vi "SelectdBaseFilesToRecover_Core.vi"(8 "Description":string="Select Condition Vector Settings To Load", 9 "Files To Recover":string[][](array[string])) -> (3 "Selected Files":string[](array[string]))   [LabVIEW 2011]
panel:
  in  "Cancel":bool caption="Trend to diagram"
  in  "OK":bool caption="Trend to diagram"
  in  "Saved settings":i32[](listbox) caption="Iznosi v èasu RS:"
  out "MP.Status parameters:":string caption="Select Files To Recover"
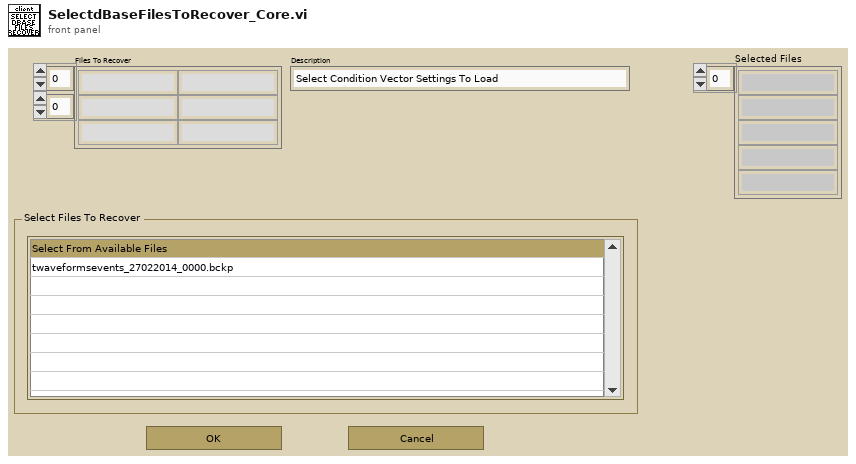
[diagram p1: front panel]
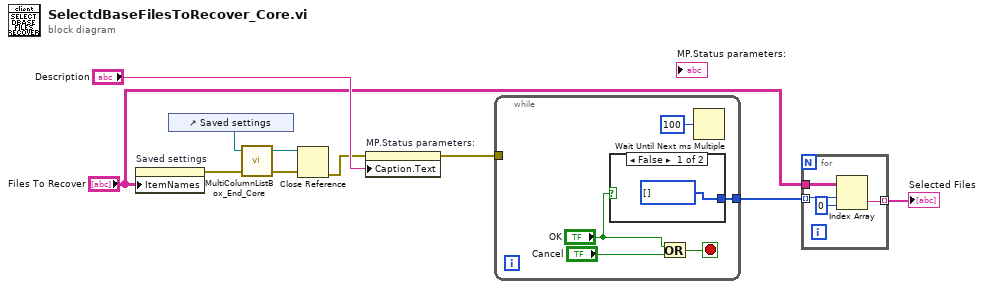
[diagram p0: block diagram]
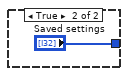
[diagram p2: hidden frame]
diagram:
  n1 = property on="Saved settings" class="MCListbox (strict)"("ItemNames"="Files To Recover") -> (error out=w9:errorcluster)  [unwired: 2 in, 1 out]
  n2 = control-ref of="Saved settings"() -> (w10:refnum<vi>)
  n3 = call "MultiColumnListBox_End_Core.vi"("error in (no error)"=w9, "MCListbox Refnum"=w10) -> ("error out"=w8:errorcluster, "MCListbox Refnum OUT"=w7:refnum<vi>)  [unwired: 2 in]
  n4 = Close Reference(reference=w7, error in (no error)=w8) -> (error out=w5:errorcluster)
  n5 = property on="MP.Status parameters:" class="Str"(error in=w5, "Caption.Text"="Description") -> (error out=w4:errorcluster)  [unwired: 1 in, 1 out]
  n6 = while {
    tunnel: [w15] -> w3
    tunnel: w4 -> [_]
    stop <- w13 stop-if-true
    n7 = case shown="False" "OK" {
      tunnel: [i32[] [] "Saved settings"] -> w15
      frame False {
      }
      frame True {
      }
    }
    n8 = Or(x="OK", y="Cancel") -> (x .or. y?=w13:bool)
    n9 = Wait Until Next ms Multiple(millisecond multiple=u32 100) -> ()  [unwired: 1 out]
  }
  n10 = for {
    tunnel: w3 -> [w19] mode=indexing
    tunnel: "Files To Recover" -> [w21]
    tunnel: [w20] -> w1 mode=indexing
    n11 = Index Array(array=w21, index (row)=w19, index (col)=0 ("disabled index (col)")) -> (element=w20:string)
  }
  "Selected Files" <- w1
